vi "LSCI332ReadSensor.vi"(0 "VISA Rsrc":refnum<visa-resource-name>="GPIB0::12::INSTR", 5 "Activées":bool[](array[boolean]) caption="Entrés Activées", 11 "error in":errorcluster) -> (4 "Données":dbl[](array[numeric]), 15 "error out":errorcluster)   [LabVIEW 2012]
doc: "Ce Vi interroge le contrôlleur de température pour la lecture en unités capteur des entrées spécifiées"
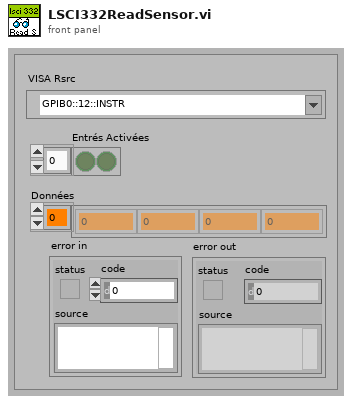
[diagram p1: front panel]
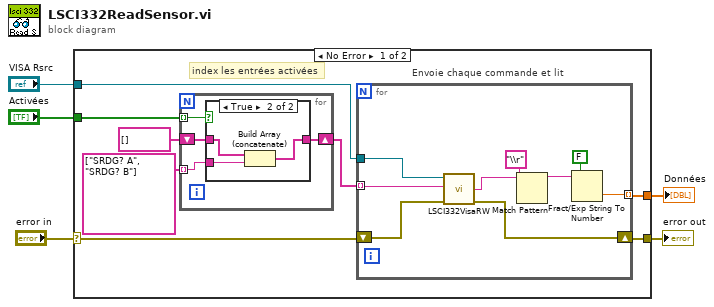
[diagram p0: block diagram]
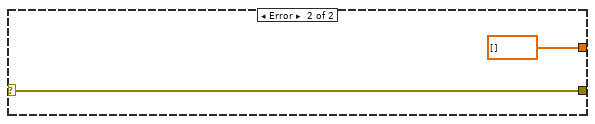
[diagram p3: hidden frame]
diagram:
  n1 = case shown="No Error" "error in" {
    selector: "error in" -> [w10 w32]
    tunnel: [w13 w32] -> w5
    tunnel: "VISA Rsrc" -> [w12 _]
    tunnel: [w11 dbl[] []] -> w3
    tunnel: "Activées" -> [w8 _]
    frame No Error {
      # "index les entrées activées"
      # "Envoie chaque commande et lit"
      n2 = for {
        tunnel: string[] ["SRDG? A", "SRDG? B"] -> [w16] mode=indexing
        tunnel: w8 -> [w17] mode=indexing
        shift-right: [w15] -> w6
        shift-left: string[] [] -> [w14]
        n3 = case shown="True" w17 {
          tunnel: w16 -> [_ w20]
          tunnel: [w18 w21] -> w15
          tunnel: w14 -> [w18 w19]
          frame False {
          }
          frame True {
            n4 = Build Array (concatenate)(w19, w20) -> (w21:string[])
          }
        }
      }
      n5 = for {
        tunnel: w6 -> [w24] mode=indexing
        shift-right: [w26] -> w13
        shift-left: w10 -> [w25]
        tunnel: w12 -> [w23]
        tunnel: [w30] -> w11 mode=indexing
        n6 = call <userlib>:"LSCI332VisaRW.vi"("error in (no error)"=w25, "ChaineCom"=w24, "VISA Rsrc"=w23) -> ("error out"=w26:errorcluster, "ChaineRep"=w22:string)  [unwired: 4 in, 2 out]
        n7 = Match Pattern(string=w22, regular expression="\\r") -> (before substring=w28:string)  [unwired: 1 in, 3 out]
        n8 = Fract/Exp String To Number(use system decimal point (T)=FALSE, string=w28) -> (number=w30:dbl)  [unwired: 2 in, 1 out]
      }
    }
    frame Error {
    }
  }
  "error out" <- w5
  "Données" <- w3
